vi "Tree Shortcut Menu Selection.vi"(6 "ItemPath":string, 8 "error in (no error)":errorcluster, 9 "Coords":T1, 10 "CtlRef":refnum<vi>, 11 "AppMgr in":refnum<class "Application Manager.lvclass">) -> (0 "error out":errorcluster, 3 "AppMgr out":refnum<class "Application Manager.lvclass">)   [LabVIEW 2017, in "Application Manager.lvclass"]
uses:
  Application Manager.lvclass
  <vilib>/Utility/miscctls.llb/LVPoint32TypeDef.ctl
  Tree Right Click Menu Data.ctl
  rql_RCM Show Message Log.ctl
  rql_RCM Show Front Panel.ctl
  rql_RCM Show Block Diagram.ctl
  rql_RCM Send Start Exiting Request.ctl
  rql_RCM Filter as Enque Worker.ctl
  rql_RCM Filter as Deque Worker.ctl
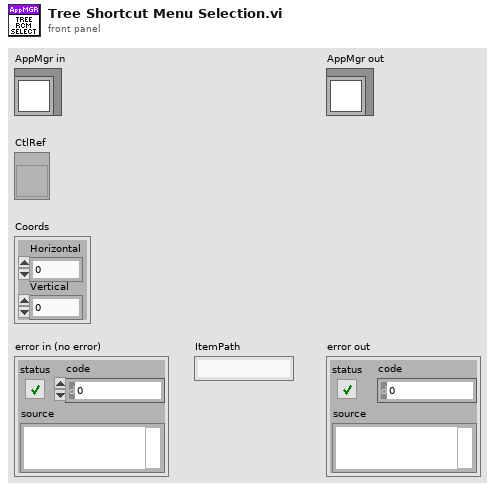
[diagram p1: front panel]
types:
  T1 = typedef "LVPoint32TypeDef.ctl" = cluster{"Horizontal":i32, "Vertical":i32}
  T2 = typedef "Application Manager.lvclass/Tree Right Click Menu Data.ctl" = cluster{"CtlRef":refnum<vi>, "Coords":T1}
  T3 = typedef "Application Manager.lvclass/rql_RCM Show Message Log.ctl" = cluster{"Tree RCM Data":T2}
  T4 = typedef "Application Manager.lvclass/rql_RCM Show Front Panel.ctl" = cluster{"Tree RCM Data":T2}
  T5 = typedef "Application Manager.lvclass/rql_RCM Show Block Diagram.ctl" = cluster{"Tree RCM Data":T2}
  T6 = typedef "Application Manager.lvclass/rql_RCM Send Start Exiting Request.ctl" = cluster{"Tree RCM Data":T2}
  T7 = typedef "Application Manager.lvclass/rql_RCM Filter as Enque Worker.ctl" = cluster{"Tree RCM Data":T2}
  T8 = typedef "Application Manager.lvclass/rql_RCM Filter as Deque Worker.ctl" = cluster{"Tree RCM Data":T2}
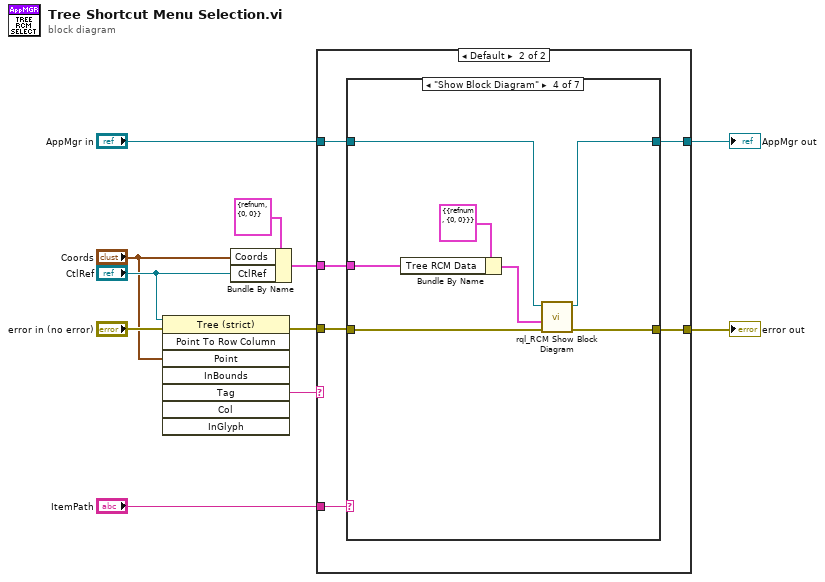
[diagram p0: block diagram]
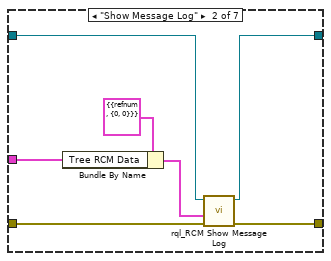
[diagram p4: hidden frame]
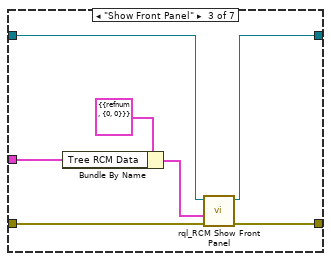
[diagram p5: hidden frame]
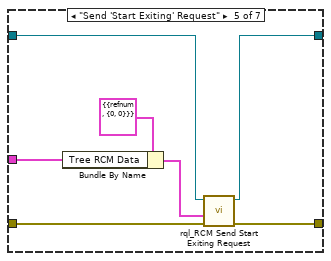
[diagram p6: hidden frame]
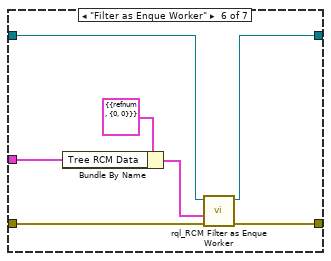
[diagram p7: hidden frame]
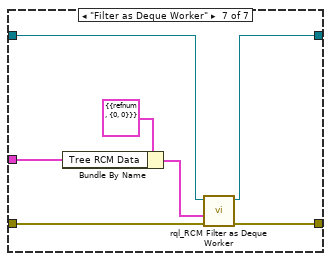
[diagram p8: hidden frame]
diagram:
  n1 = invoke class="Tree (strict)" method="Point To Row Column"(reference="CtlRef", error in="error in (no error)", "Point"="Coords") -> (error out=w3:errorcluster, "Tag"=w1:string)  [unwired: 5 in, 6 out]
  n2 = Bundle By Name(cluster=T2 {"CtlRef"=refnum, "Coords"={"Horizontal"=0, "Vertical"=0}} ("Tree RCM Data"), "Coords"="Coords", "CtlRef"="CtlRef") -> (w6:T2)
  n3 = case shown="Default" w1 {
    tunnel: [w12 w19] -> w11
    tunnel: "AppMgr in" -> [w12 w18]
    tunnel: [w13 w17] -> w9
    tunnel: w6 -> [_ w16]
    tunnel: "ItemPath" -> [_ w15]
    tunnel: w3 -> [w13 w14]
    frame "" {
      # "right click activated over white space.\nignore."
    }
    frame Default {
      n4 = case shown="\"Show Block Diagram\"" w15 {
        tunnel: [w21 w28 w35 w42 w49 w56 w63] -> w19
        tunnel: w18 -> [w21 w27 w34 w41 w48 w55 w62]
        tunnel: [w20 w26 w33 w40 w47 w54 w61] -> w17
        tunnel: w14 -> [w20 w25 w32 w39 w46 w53 w60]
        tunnel: w16 -> [_ w22 w29 w36 w43 w50 w57]
        frame Default {
        }
        frame "Show Message Log" {
          n5 = Bundle By Name(cluster=T3 {"Tree RCM Data"={"CtlRef"=refnum, "Coords"={"Horizontal"=0, "Vertical"=0}}} ("Data in"), "Tree RCM Data"=w22) -> (w23:T3)
          n6 = call "rql_RCM Show Message Log.vi"("error in"=w25, "Data in"=w23, "Application Manager in"=w27) -> ("error out"=w26:errorcluster, "dup Application Manager out"=w28:refnum<class "Application Manager.lvclass">)  [unwired: 7 in]
        }
        frame "Show Front Panel" {
          n7 = Bundle By Name(cluster=T4 {"Tree RCM Data"={"CtlRef"=refnum, "Coords"={"Horizontal"=0, "Vertical"=0}}} ("Data in"), "Tree RCM Data"=w29) -> (w30:T4)
          n8 = call "rql_RCM Show Front Panel.vi"("error in"=w32, "Data in"=w30, "Application Manager in"=w34) -> ("error out"=w33:errorcluster, "dup Application Manager out"=w35:refnum<class "Application Manager.lvclass">)  [unwired: 7 in]
        }
        frame "Show Block Diagram" {
          n9 = Bundle By Name(cluster=T5 {"Tree RCM Data"={"CtlRef"=refnum, "Coords"={"Horizontal"=0, "Vertical"=0}}} ("Data in"), "Tree RCM Data"=w36) -> (w37:T5)
          n10 = call "rql_RCM Show Block Diagram.vi"("error in"=w39, "Data in"=w37, "Application Manager in"=w41) -> ("error out"=w40:errorcluster, "dup Application Manager out"=w42:refnum<class "Application Manager.lvclass">)  [unwired: 7 in]
        }
        frame "Send 'Start Exiting' Request" {
          n11 = Bundle By Name(cluster=T6 {"Tree RCM Data"={"CtlRef"=refnum, "Coords"={"Horizontal"=0, "Vertical"=0}}} ("Data in"), "Tree RCM Data"=w43) -> (w44:T6)
          n12 = call "rql_RCM Send Start Exiting Request.vi"("error in"=w46, "Data in"=w44, "Application Manager in"=w48) -> ("error out"=w47:errorcluster, "dup Application Manager out"=w49:refnum<class "Application Manager.lvclass">)  [unwired: 7 in]
        }
        frame "Filter as Enque Worker" {
          n13 = Bundle By Name(cluster=T7 {"Tree RCM Data"={"CtlRef"=refnum, "Coords"={"Horizontal"=0, "Vertical"=0}}} ("Data in"), "Tree RCM Data"=w50) -> (w51:T7)
          n14 = call "rql_RCM Filter as Enque Worker.vi"("error in"=w53, "Data in"=w51, "Application Manager in"=w55) -> ("error out"=w54:errorcluster, "dup Application Manager out"=w56:refnum<class "Application Manager.lvclass">)  [unwired: 7 in]
        }
        frame "Filter as Deque Worker" {
          n15 = Bundle By Name(cluster=T8 {"Tree RCM Data"={"CtlRef"=refnum, "Coords"={"Horizontal"=0, "Vertical"=0}}} ("Data in"), "Tree RCM Data"=w57) -> (w58:T8)
          n16 = call "rql_RCM Filter as Deque Worker.vi"("error in"=w60, "Data in"=w58, "Application Manager in"=w62) -> ("error out"=w61:errorcluster, "dup Application Manager out"=w63:refnum<class "Application Manager.lvclass">)  [unwired: 7 in]
        }
      }
    }
  }
  "AppMgr out" <- w11
  "error out" <- w9
